vi "subCleanUpDependencies.vi"(8 "error in (no error)":errorcluster, 11 "SolutionBuilder in":refnum<class "SolutionBuilder.lvclass">) -> (0 "error out":errorcluster, 3 "SolutionBuilder out":refnum<class "SolutionBuilder.lvclass">)   [LabVIEW 2019, in "SolutionBuilder.lvlib" / "SolutionBuilder.lvclass"]
uses:
  SolutionBuilder.lvclass
  SolutionBuilder.lvclass/SolutionBuilder.ctl
  ProjectItem/ProjectItem.lvclass
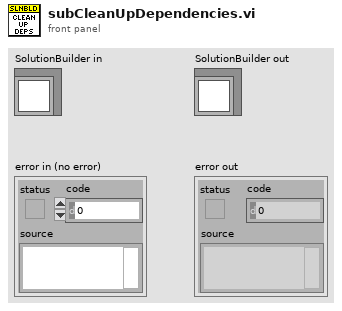
[diagram p1: front panel]
types:
  T1 = typedef "SolutionBuilder.lvlib/SolutionBuilder.lvclass/ProjectItemMap.ctl" = map{path, refnum<class "ProjectItem.lvclass">[]}
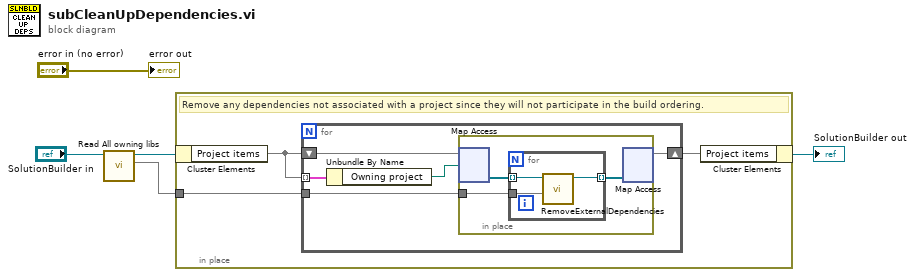
[diagram p0: block diagram]
diagram:
  n1 = call-dynamic "Read All owning libs.vi"("SolutionBuilder in"="SolutionBuilder in") -> ("All owning libs"=w1:set{string}, "SolutionBuilder out"=w2:refnum<class "SolutionBuilder.lvclass">)  [unwired: 9 in]
  n2 = in-place {
    in-place-border: w1 -> [w7]
    # "Remove any dependencies not associated with a project since they will not participate in the build ordering."
    n3 = in-place-cluster #1(w2) -> ("Project items"=w8:T1)
    n4 = for {
      tunnel: w8 -> [w13] mode=indexing
      shift-right: [w9] -> w6
      shift-left: w8 -> [w11]
      tunnel: w7 -> [w10]
      n5 = Unbundle By Name(w13) -> ("Owning project"=w12:path)
      n6 = in-place {
        in-place-border: w10 -> [w15]
        n7 = in-place-map #2(w11, w12) -> (w16:refnum<class "ProjectItem.lvclass">[])  [unwired: 1 in, 1 out]
        n8 = for {
          tunnel: w16 -> [w19] mode=indexing
          tunnel: w15 -> [w18]
          tunnel: [w17] -> w14 mode=indexing
          n9 = call-dynamic "RemoveExternalDependencies.vi"("Possible deps"=w18, "ProjectItem in"=w19) -> ("ProjectItem out"=w17:refnum<class "ProjectItem.lvclass">)  [unwired: 8 in, 1 out]
        }
        n10 = in-place-map #2(w14) -> (w9:T1)  [unwired: 1 in, 2 out]
      }
    }
    n11 = in-place-cluster #1("Project items"=w6) -> (→"SolutionBuilder out":refnum<class "SolutionBuilder.lvclass">)
  }
  "error out" <- "error in (no error)"
